vi "ROI entry-User ROI event-Apply new ROI.vi"(8 "error in (no error)":errorcluster, 10 "Input cluster":T1 {"ROIs Info []"."FOV" min=1.0 max=10.0 step=1.0; "ROIs Info []"."Frame Size" min=1.0 max=10.0 step=1.0; "ROIs Info []"."Laser Power" min=1.0 max=10.0 step=0.10000000149011612; "ROIs Info []"."Rel. Resolution" min=1.0 max=10.0 step=1.0; "ROIs Info []"."POI Dwell time" min=1.0 max=10.0 step=0.10000000149011612; "ROIs Info []"."Zoom" min=1.0 max=10.0 step=0.10000000149011612; "Last Image Display Event info"."Tool" items=["None", "Selection Tool", "Point Tool", "Line Tool", "Rectangle Tool", "Oval Tool", "Polygon Tool", "ClosedFreehandTool", "Annulus Tool", "Rotated Rectangle Tool", "Zoom Tool", "Pan Tool", "Polyline Tool", "Freehand Tool"]; "Last Image Display Event info"."Type" items=["No Event"=0, "Click Event"=1, "Draw Event"=2, "Size Event"=4, "Scroll Event"=5, "Double Click Event"=8]}) -> (0 "error IO":errorcluster)   [LabVIEW 2020]
uses:
  Typedefs/ROI Entry screen VI interface 1.ctl
  Typedefs/Last Image Display Event info.ctl
  Typedefs/ROI spec.ctl
  Typedefs/ROI ID Enum.ctl
  Typedefs/ROI management FG states.ctl
  ROI Entry screen/Globals/gl_ROI Entry UI globals.vi
panel:
  out "Last valid":T1 {"ROIs Info []"."FOV" min=1.0 max=10.0 step=1.0; "ROIs Info []"."Frame Size" min=1.0 max=10.0 step=1.0; "ROIs Info []"."Laser Power" min=1.0 max=10.0 step=0.10000000149011612; "ROIs Info []"."Rel. Resolution" min=1.0 max=10.0 step=1.0; "ROIs Info []"."POI Dwell time" min=1.0 max=10.0 step=0.10000000149011612; "ROIs Info []"."Zoom" min=1.0 max=10.0 step=0.10000000149011612; "Last Image Display Event info"."Tool" items=["None", "Selection Tool", "Point Tool", "Line Tool", "Rectangle Tool", "Oval Tool", "Polygon Tool", "ClosedFreehandTool", "Annulus Tool", "Rotated Rectangle Tool", "Zoom Tool", "Pan Tool", "Polyline Tool", "Freehand Tool"]; "Last Image Display Event info"."Type" items=["No Event"=0, "Click Event"=1, "Draw Event"=2, "Size Event"=4, "Scroll Event"=5, "Double Click Event"=8]}
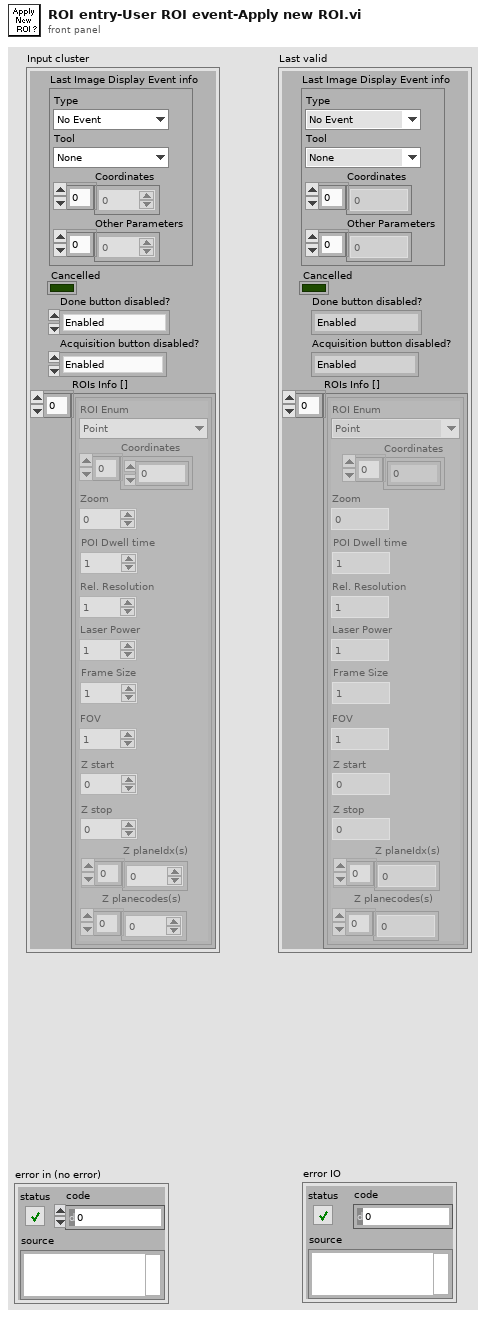
[diagram p1: front panel]
types:
  T1 = typedef "ROI Entry screen VI interface 1.ctl" = cluster{"Last Image Display Event info":T2, "ROIs Info []":T3[], "Cancelled":bool, "Done button disabled?":enum8{"Enabled", "Disabled", "Disabled and Grayed Out"}, "Acquisition button disabled?":enum8{"Enabled", "Disabled", "Disabled and Grayed Out"}}
  T2 = typedef "Last Image Display Event info.ctl" = cluster{"Type":i32, "Tool":i32, "Coordinates":i32[], "Other Parameters":sgl[]}
  T3 = typedef "ROI spec.ctl" = cluster{"ROI Enum":T4, "Coordinates":i32[], "Zoom":dbl, "POI Dwell time":dbl, "Rel. Resolution":dbl, "Laser Power":dbl, "Frame Size":dbl, "FOV":dbl, "Z start":dbl, "Z stop":dbl, "Z planeIdx(s)":i32[], "Z planecodes(s)":u8[]}
  T4 = typedef "ROI ID Enum.ctl" = enum16{"Point", "MiniScan", "Comp. MiniScan", "Rectangle", "Comp. volume", "Arb. plane point", "None"}
  T5 = typedef "ROI management FG states.ctl" = enum16{"Read", "Write", "Write-from dataset", "Clear Last", "Clear All", "Delete ROI", "Update ROIs time", "Reload last ROI set", "Modify ROI Parameters", "Offset all ROI", "Offset visible ROI", "Modify Dwell Time", "Modify Laser Power"}
  T6 = typedef "ROI entry screen ctrl refs cluster.ctl" = cluster{"Done button":refnum<vi>, "Imaging button":refnum<vi>, "Acquisition button":refnum<vi>, "Scan dwell time per pixel (us)":refnum<vi>, "# of planes":refnum<vi>, "Zoom Ctrl":refnum<vi>, "Equal size":refnum<vi>, "Channel":refnum<vi>, "Image Display":refnum<vi>, "Z-Plane Selector":refnum<vi>, "Number of lines left":refnum<vi>, "Z-stack folder path":refnum<vi>, "POI Density":refnum<vi>, "Arb Plane Entry":refnum<vi>, "Whole Plane":refnum<vi>, "Line Mode":refnum<vi>, "Clear Last":refnum<vi>, "Clear All":refnum<vi>, "Delete Lines":refnum<vi>, "Trial Length (sec)":refnum<vi>, "Palette Type":refnum<vi>, "Intensity slider":refnum<vi>, "# POI":refnum<vi>, "Max Z Proj":refnum<vi>, "Zplane ind":refnum<vi>, "Wavelength (nm)":refnum<vi>, "Number of Trials":refnum<vi>, "Funct stim.trig.enable":refnum<vi>, "Funct stim.trig.delay (s)":refnum<vi>, "Line Mode":refnum<vi>, "Step size (µm)":refnum<vi>, "ROI move mode":refnum<vi>, "Cool-down time (s)":refnum<vi>, "Enable cool-down time":refnum<vi>, "Motor Z ind. (um)":refnum<vi>, "AOL Z ind. (um)":refnum<vi>, "Load Reference Image":refnum<vi>, "Rel.  Res.":refnum<vi>, "ROI LIST":refnum<vi>, "Show All":refnum<vi>, "ROI Type":refnum<vi>, "Start Plane":refnum<vi>, "Stop Plane":refnum<vi>, "Offset ROI":refnum<vi>, "Tab Control":refnum<vi>, "Laser Power(%)":refnum<vi>, "Cycle rate":refnum<vi>, "FOV (Ind.)":refnum<vi>, "Frame Size (Ind.)":refnum<vi>, "Resolution (Ind.)":refnum<vi>, "Pixel Density (Ind)":refnum<vi>, "Laser Power (Ind.)":refnum<vi>, "Dwell Time (Ind.)":refnum<vi>, "Adj MC":refnum<vi>}
  T7 = typedef "Redraw ROI.ctl" = enum16{"Redraw All", "Redraw Deselected", "Draw Last", "Redraw Selected"}
  T8 = enum8{"Enabled", "Disabled", "Disabled and Grayed Out"}
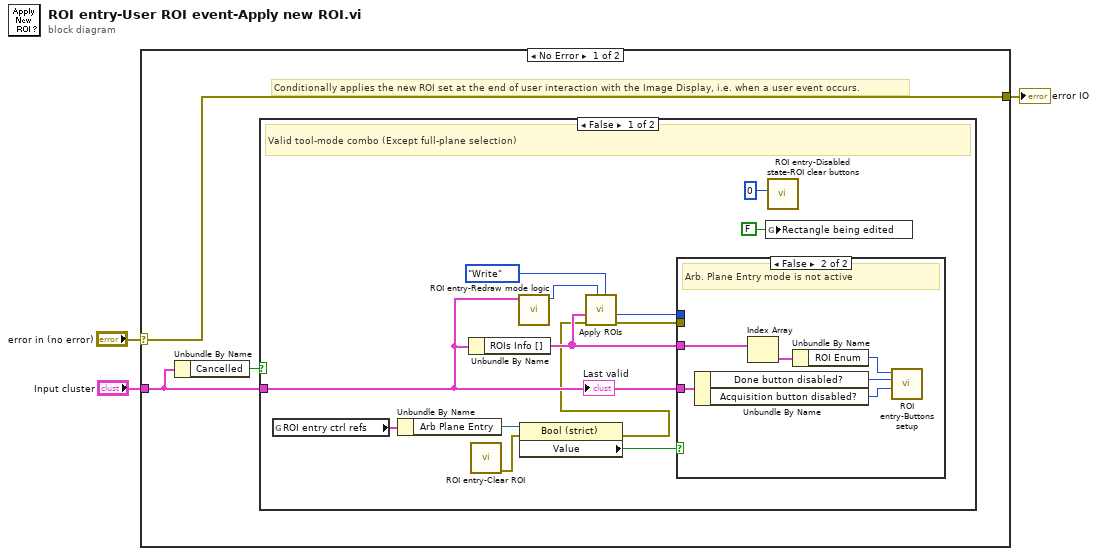
[diagram p0: block diagram]
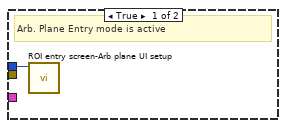
[diagram p2: hidden frame]
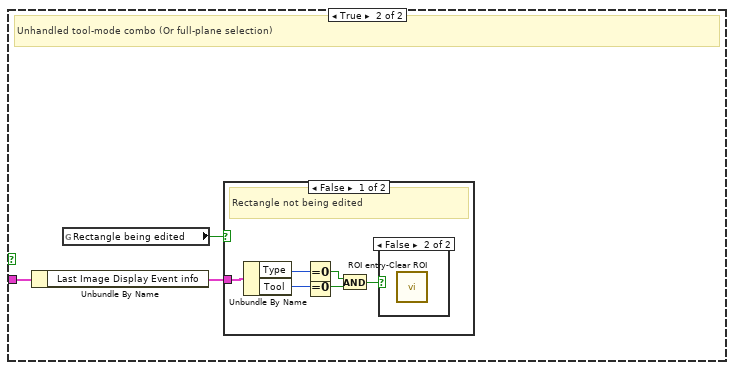
[diagram p3: hidden frame]
diagram:
  n1 = case shown="No Error" "error in (no error)" {
    selector: "error in (no error)" -> [w4 w36]
    tunnel: "Input cluster" -> [w6 _]
    tunnel: [w4 w36] -> w1
    frame No Error {
      # "Conditionally applies the new ROI set at the end of user interaction with the Image Display, i.e. when a user event occurs."
      n2 = Unbundle By Name(w6) -> ("Cancelled"=w5:bool)
      n3 = case shown="False" w5 {
        tunnel: w6 -> [w13 w28]
        frame False {
          # "Valid tool-mode combo (Except full-plane selection)"
          n4 = global read "gl_ROI Entry UI globals.vi" "ROI entry ctrl refs"() -> (w17:T6)
          n5 = Unbundle By Name(w17) -> ("Arb Plane Entry"=w18:refnum<vi>)
          n6 = Unbundle By Name(w13) -> ("ROIs Info []"=w14:T3[])
          n7 = call "ROI entry-Clear ROI.vi"() -> ("error out"=w11:errorcluster)  [unwired: 11 in]
          n8 = call "ROI entry-Redraw mode logic.vi"("Input cluster"=w13) -> ("Mode"=w15:T7)  [unwired: 10 in]
          n9 = property class="Bool (strict)"(reference=w18, error in=w11) -> (error out=w12:errorcluster, "Value"=w16:bool)  [unwired: 1 out]
          n10 = call "Apply ROIs.vi"("Function"=ROI_management_FG_states."Write", "Mode (Redraw All)"=w15, "error in (no error)"=w12, "ROIs Info []"=w14) -> ("error out"=w7:errorcluster, "Number of ROI"=w19:i32)  [unwired: 5 in, 1 out]
          n11 = case shown="False" w16 {
            tunnel: w14 -> [_ w26]
            tunnel: w19 -> [w20 _]
            tunnel: w7 -> [_ _]
            tunnel: w13 -> [_ w23]
            frame True {
              # "Arb. Plane Entry mode is active"
              n12 = call "ROI entry screen-Arb plane UI setup.vi"("Number of ROI"=w20) -> ()  [unwired: 11 in]
            }
            frame False {
              # "Arb. Plane Entry mode is not active"
              n13 = Unbundle By Name(w23) -> ("Done button disabled?"=w22:T8, "Acquisition button disabled?"=w21:T8)
              n14 = Index Array(array=w26) -> (element=w25:T3)  [unwired: 1 in]
              n15 = Unbundle By Name(w25) -> ("ROI Enum"=w24:T4)
              n16 = call "ROI entry-Buttons setup.vi"("Acquisition button disabled?"=w21, "Done button disabled?"=w22, "ROI Enum"=w24) -> ()  [unwired: 9 in]
            }
          }
          n17 = global write "gl_ROI Entry UI globals.vi" "Rectangle being edited"(FALSE ("Rectangle being edited")) -> ()
          n18 = call "ROI entry-Disabled state-ROI clear buttons.vi"("State"=0) -> ()  [unwired: 10 in, 1 out]
          "Last valid" <- w13
        }
        frame True {
          # "Unhandled tool-mode combo (Or full-plane selection)"
          n19 = Unbundle By Name(w28) -> ("Last Image Display Event info"=w27:T2)
          n20 = global read "gl_ROI Entry UI globals.vi" "Rectangle being edited"() -> (w29:bool)
          n21 = case shown="False" w29 {
            tunnel: w27 -> [w32 _]
            frame False {
              # "Rectangle not being edited"
              n22 = Unbundle By Name(w32) -> ("Type"=w31:i32, "Tool"=w30:i32)
              n23 = Equal To 0?(x=w31) -> (x = 0?=w35:bool)
              n24 = Equal To 0?(x=w30) -> (x = 0?=w34:bool)
              n25 = And(x=w35, y=w34) -> (x .and. y?=w33:bool)
              n26 = case shown="False" w33 {
                frame True {
                }
                frame False {
                  n27 = call "ROI entry-Clear ROI.vi"() -> ()  [unwired: 11 in, 1 out]
                }
              }
            }
            frame True {
              # "Retains the NI ROI box\nto allow the user rotate it/edit it\nbefore accepting it."
              # "Rectangle being edited"
            }
          }
        }
      }
    }
    frame Error {
    }
  }
  "error IO" <- w1
